vi "Send TX Message.vi"(8 "error in (no error)":errorcluster, 11 "RxTx in":refnum<class "RxTx.lvclass">) -> (0 "error out":errorcluster, 3 "RxTx out":refnum<class "RxTx.lvclass">)   [LabVIEW 2018, in "RxTx.lvclass"]
uses:
  RxTx.lvclass
  RxTx.lvclass/RxTx.ctl
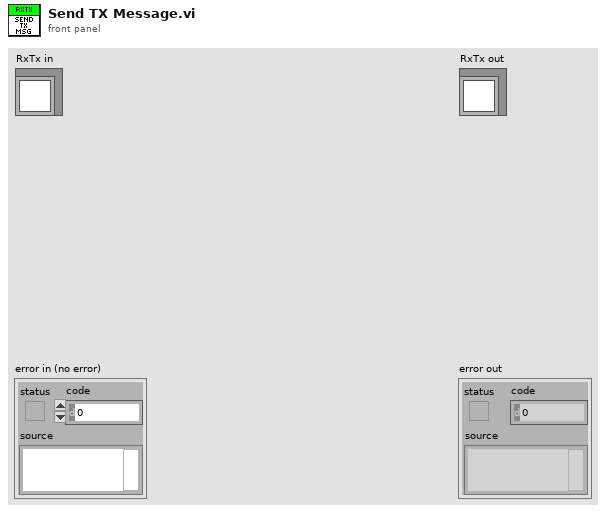
[diagram p1: front panel]
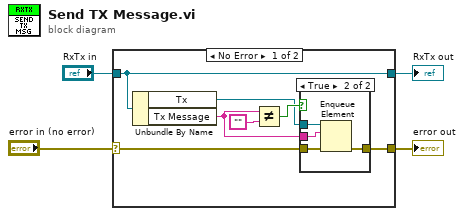
[diagram p0: block diagram]
diagram:
  n1 = case shown="No Error" "error in (no error)" {
    selector: "error in (no error)" -> [w6 w18]
    tunnel: [w5 w18] -> w3
    tunnel: [w11 w17] -> w1
    tunnel: "RxTx in" -> [w11 w17]
    frame No Error {
      n2 = Unbundle By Name(w11) -> ("Tx"=w8:refnum<queue>, "Tx Message"=w7:string)
      n3 = Not Equal?(x=w7, y="") -> (x != y?=w9:bool)
      n4 = case shown="True" w9 {
        tunnel: w8 -> [_ w16]
        tunnel: w7 -> [_ w15]
        tunnel: w6 -> [w12 w14]
        tunnel: [w12 w13] -> w5
        frame False {
        }
        frame True {
          n5 = Enqueue Element(queue=w16, element=w15, error in (no error)=w14) -> (error out=w13:errorcluster)  [unwired: 1 in, 2 out]
        }
      }
    }
    frame Error {
    }
  }
  "error out" <- w3
  "RxTx out" <- w1
